vi "Image Display Zoom to Fit.vi"(8 "Error In":errorcluster, 9 "Keep Aspect Ratio (T)":bool=TRUE, 11 "Display Image Control Refnum":T1) -> (0 "Error Out":errorcluster)   [LabVIEW 2021, in "Image.lvlib"]
uses:
  Image Control Refnum.ctl
  Image.lvlib
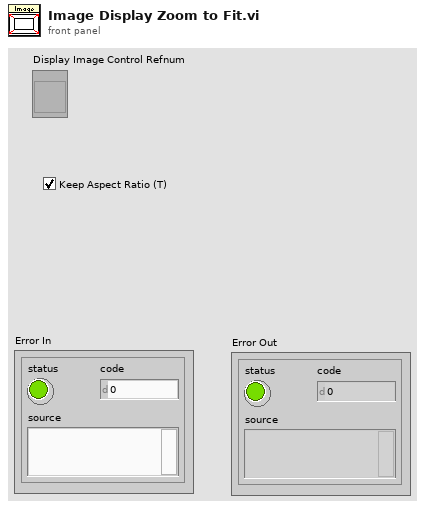
[diagram p1: front panel]
types:
  T1 = typedef "Image.lvlib/Image Control Refnum.ctl" = refnum<vi>
  T2 = typedef "IMAQ Image.ctl" = refnum<image>
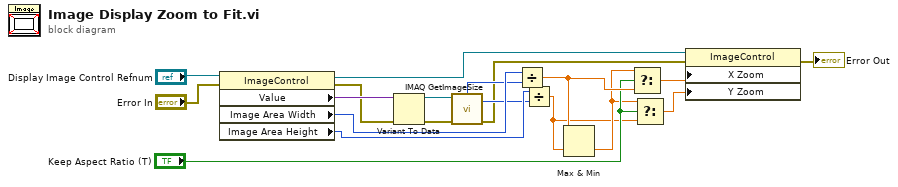
[diagram p0: block diagram]
diagram:
  n1 = property class="ImageControl"(reference="Display Image Control Refnum", error in="Error In") -> (reference out=w8:T1, error out=w16:errorcluster, "Value"=w17:variant, "Image Area Width"=w13:u32, "Image Area Height"=w11:u32)
  n2 = Variant To Data(error in=w16, Variant=w17) -> (data=w15:T2, error out=w14:errorcluster)  [unwired: 1 in]
  n3 = call "IMAQ GetImageSize"("Image"=w15, "error in (no error)"=w14) -> ("Y Resolution"=w10:i32, "X Resolution"=w12:i32, "error out"=w9:errorcluster)  [unwired: 2 in]
  n4 = Divide(x=w13, y=w12) -> (x/y=w6:dbl)
  n5 = Divide(x=w11, y=w10) -> (x/y=w3:dbl)
  n6 = Max & Min(x=w6, y=w3) -> (min(x,y)=w4:dbl)  [unwired: 1 out]
  n7 = Select(t=w4, s="Keep Aspect Ratio (T)", f=w6) -> (s? t:f=w2:dbl)
  n8 = Select(t=w4, s="Keep Aspect Ratio (T)", f=w3) -> (s? t:f=w1:dbl)
  n9 = property class="ImageControl"(reference=w8, error in=w9, "X Zoom"=w2, "Y Zoom"=w1) -> (error out=→"Error Out":errorcluster)  [unwired: 1 out]
